vi "gu_string_to_codepoint_array.vi"(8 "error in":errorcluster, 11 "Encoded String":T1) -> (0 "error out":errorcluster, 3 "Codepoint Array":i32[](array[numeric]) format="%04x")   [LabVIEW 2020, in "G-Unicode.lvlib"]
uses:
  G-Unicode.lvlib
  Types/Encoded UTF-8 String.ctl
  5c793459-c97f-49eb-b871-f007f412847a.vi
  gu_free.vi
  5c793459-c97f-49eb-b871-f007f412847a.vi/bf7dd0c3-7326-468c-a5c4-9eb034008d84.vi
  <vilib>/Utility/error.llb/Error Cluster From Error Code.vi
  lib/g_unicode_32.dll
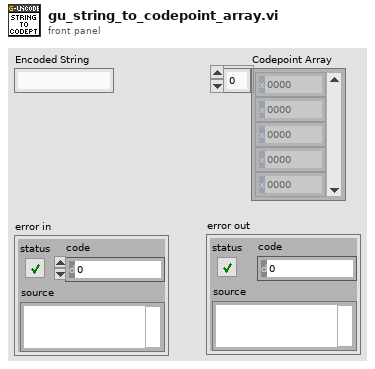
[diagram p1: front panel]
types:
  T1 = typedef "G-Unicode.lvlib/Encoded UTF-8 String.ctl" = string
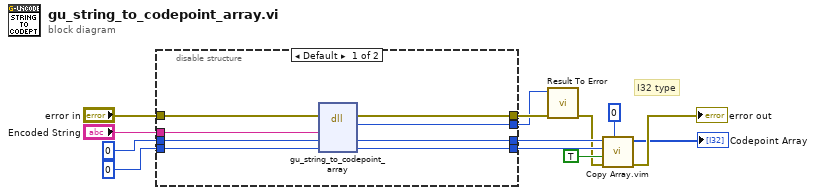
[diagram p0: block diagram]
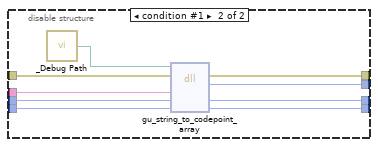
[diagram p2: hidden frame]
diagram:
  # "I32 type"
  n1 = disable-structure shown="Default" {
    disable-tunnel: "Encoded String" -> [w20 w29]
    disable-tunnel: "error in" -> [w21 w30]
    disable-tunnel: [w19 w28] -> w11
    disable-tunnel: [w18 w27] -> w9
    disable-tunnel: [w17 w26] -> w8
    disable-tunnel: [w16 w24] -> w10
    disable-tunnel: i64 0 ("codepoint_array") -> [w15 w23]
    disable-tunnel: 0 ("codepoint_array_size") -> [w14 w22]
    frame condition #0 (active) {
      n2 = dll-call lib="C:/github/dataflowg/g-unicode/src/LabVIEW/G-Unicode/lib/g_unicode_*.*" fn="gu_string_to_codepoint_array"(error in=w21, "string"=w20, "codepoint_array"=w15, "codepoint_array_size"=w14) -> (error out=w19:errorcluster, "result"=w16:i32, "codepoint_array"=w18:i64, "codepoint_array_size"=w17:i32)  [unwired: 3 in, 1 out]
    }
    frame condition #1 {
      n3 = call "_Debug Path.vi"() -> ("Debug Path"=w25:path)
      n4 = dll-call lib="?" fn="gu_string_to_codepoint_array"(path in=w25, error in=w30, "string"=w29, "codepoint_array"=w23, "codepoint_array_size"=w22) -> (error out=w28:errorcluster, "result"=w24:i32, "codepoint_array"=w27:i64, "codepoint_array_size"=w26:i32)  [unwired: 2 in, 1 out]
    }
  }
  n5 = call "Result To Error.vi"("error in (no error)"=w11, "Result Code"=w10) -> ("error out"=w5:errorcluster)  [unwired: 9 in]
  n6 = call "Copy Array.vim"("Type"=0, "error in"=w5, "free (F)"=TRUE, "size"=w8, "pointer"=w9) -> ("error out"=→"error out":errorcluster, "array"=→"Codepoint Array":i32[])  [unwired: 5 in]
